vi "Destroy.vi"(8 "error in":errorcluster, 11 "Potting Procedure in":refnum<class "Potting Procedure.lvclass">) -> (0 "error out":errorcluster)   [LabVIEW 2011, in "Potting Procedure.lvclass"]
uses:
  Potting Procedure.lvclass
  Potting Procedure.lvclass/Potting Procedure.ctl
  Shared Components/Gantry Class/Gantry Class.lvclass
  Shared Components/Config Manager Class/Config Manager Class.lvclass
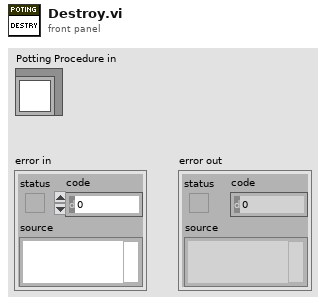
[diagram p1: front panel]
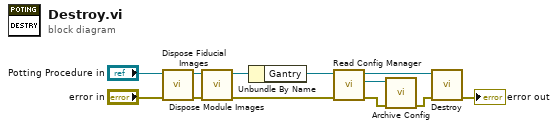
[diagram p0: block diagram]
diagram:
  n1 = call-dynamic "Dispose Fiducial Images.vi"("error in"="error in", "Potting Procedure in"="Potting Procedure in") -> ("error out"=w11:errorcluster, "Potting Procedure out"=w10:refnum<class "Potting Procedure.lvclass">)  [unwired: 8 in]
  n2 = call-dynamic "Dispose Module Images.vi"("error in"=w11, "Potting Procedure in"=w10) -> ("error out"=w4:errorcluster, "Potting Procedure out"=w8:refnum<class "Potting Procedure.lvclass">)  [unwired: 8 in]
  n3 = Unbundle By Name(w8) -> ("Gantry"=w6:refnum<class "Gantry Class.lvclass">)
  n4 = call-dynamic "Read Config Manager.vi"("error in"=w4, "Gantry in"=w6) -> ("error out"=w3:errorcluster, "Config Manager"=w5:refnum<class "Config Manager Class.lvclass">, "Gantry out"=w2:refnum<class "Gantry Class.lvclass">)  [unwired: 7 in]
  n5 = call "Archive Config.vi"("error in"=w3, "Config Manager in"=w5) -> ("error out"=w1:errorcluster)  [unwired: 8 in, 1 out]
  n6 = call "Destroy.vi"("error in"=w1, "Gantry Class in"=w2) -> ("error out"=→"error out":errorcluster)  [unwired: 9 in]
